vi "Lab Panel V5.0.vi"() -> ()   [LabVIEW 2013] (continued)
                  tunnel: w3944 -> [_ _ _ w4028 _]
                  tunnel: w3943 -> [_ _ _ w4027 _]
                  tunnel: w3942 -> [_ _ _ w4026 _]
                  tunnel: w3941 -> [_ _ _ w4025 _]
                  tunnel: w3940 -> [_ _ _ w4024 _]
                  tunnel: w3939 -> [_ _ _ w4023 _]
                  tunnel: w3938 -> [_ _ _ w4022 _]
                  frame #0 {
                    n2306 = Merge Signals(w3998, w3997, w3996, w3995, w3994, w3993, w3992, w3991, w3990, w3989) -> (→"TEST AMPS CHART":dynamicdata)
                  }
                  frame #1 {
                    n2307 = Merge Signals(w4009, w4008, w4007, w4006, w4005, w4004, w4003, w4002, w4001, w4000) -> (→"TEST VOLTS CHART":dynamicdata)
                  }
                  frame #2 {
                    n2308 = Merge Signals(w4020, w4019, w4018, w4017, w4016, w4015, w4014, w4013, w4012, w4011) -> (→"TEMPERATURE (L) CHART":dynamicdata)
                  }
                  frame #3 {
                    n2309 = Merge Signals(w4031, w4030, w4029, w4028, w4027, w4026, w4025, w4024, w4023, w4022) -> (→"TEMPERATURE (N) CHART":dynamicdata)
                  }
                  frame #4 {
                    n2310 = local read "TEMPERATURE (N) CHART"() -> (w4032:dynamicdata)
                    n2311 = local read "TEMPERATURE (L) CHART"() -> (w4033:dynamicdata)
                    n2312 = local read "TEST VOLTS CHART"() -> (w4034:dynamicdata)
                    n2313 = local read "TEST AMPS CHART"() -> (w4035:dynamicdata)
                    n2314 = global write "Global display 3.vi" "graph temp N"(w4032) -> ()
                    n2315 = global write "Global display 3.vi" "graph temp L"(w4033) -> ()
                    n2316 = global write "Global display 3.vi" "graph volts"(w4034) -> ()
                    n2317 = global write "Global display 3.vi" "graph amps"(w4035) -> ()
                  }
                }
              }
            }
          }
          frame #14 {
            # "check for amps fail"
            # "check for cycle test & temperature rise fail conditions"
            n2318 = local read "on loops"() -> (w4062:dbl)
            n2319 = local read "jig cycle"() -> (w4059:dbl)
            n2320 = local read "jig cycle"() -> (w4064:dbl)
            n2321 = Add(x=w4062, y=3.0) -> (x+y=w4060:dbl)
            n2322 = Equal?(x=w4059, y=w4060) -> (x = y?=w4055:bool)
            n2323 = local read "Fail Loops"() -> (w4036:dbl)
            n2324 = Equal?(x=w4064, y=1.0) -> (x = y?=w4057:bool)
            n2325 = global write "Global 1.vi" "fail count"(w4036) -> ()
            n2326 = stacked-sequence {
              tunnel: w4058 -> [w4067 _ _ _ _ _ _ _ _ _]
              tunnel: w4057 -> [w4068 w4088 w4108 w4128 w4148 w4168 w4188 w4208 w4228 w4248]
              tunnel: w4056 -> [w4065 _ _ _ _ _ _ _ _ _]
              tunnel: w4055 -> [w4066 w4087 w4107 w4127 w4147 w4167 w4187 w4207 w4227 w4247]
              tunnel: w4054 -> [_ w4086 _ _ _ _ _ _ _ _]
              tunnel: w4053 -> [_ w4085 _ _ _ _ _ _ _ _]
              tunnel: w4052 -> [_ _ w4106 _ _ _ _ _ _ _]
              tunnel: w4051 -> [_ _ w4105 _ _ _ _ _ _ _]
              tunnel: w4050 -> [_ _ _ w4126 _ _ _ _ _ _]
              tunnel: w4049 -> [_ _ _ w4125 _ _ _ _ _ _]
              tunnel: w4048 -> [_ _ _ _ w4146 _ _ _ _ _]
              tunnel: w4047 -> [_ _ _ _ w4145 _ _ _ _ _]
              tunnel: w4046 -> [_ _ _ _ _ w4166 _ _ _ _]
              tunnel: w4045 -> [_ _ _ _ _ w4165 _ _ _ _]
              tunnel: w4044 -> [_ _ _ _ _ _ w4186 _ _ _]
              tunnel: w4043 -> [_ _ _ _ _ _ w4185 _ _ _]
              tunnel: w4042 -> [_ _ _ _ _ _ _ w4206 _ _]
              tunnel: w4041 -> [_ _ _ _ _ _ _ w4205 _ _]
              tunnel: w4040 -> [_ _ _ _ _ _ _ _ w4226 _]
              tunnel: w4039 -> [_ _ _ _ _ _ _ _ w4225 _]
              tunnel: w4038 -> [_ _ _ _ _ _ _ _ _ w4246]
              tunnel: w4037 -> [_ _ _ _ _ _ _ _ _ w4245]
              frame #0 {
                # "LAB01-1"
                n2327 = case shown="True" w4065 {
                  tunnel: w4068 -> [_ w4081]
                  tunnel: w4067 -> [_ w4078]
                  tunnel: w4066 -> [_ w4077]
                  frame False {
                  }
                  frame True {
                    n2328 = local read "TEMP START LAB01-1"() -> (w4083:cluster{"TL":dbl, "TN":dbl})
                    n2329 = local read "RESULT LAB01-1"() -> (w4072:bool)
                    n2330 = local read "FAIL LAB01-1"() -> (w4075:cluster{"LO":dbl, "HI":dbl})
                    n2331 = local read "TDMS LAB01-1"() -> (w4082:refnum<k34>)
                    n2332 = local read "SET LAB01-1"() -> (w4079:T5)
                    n2333 = local read "DISP LAB01-1"() -> (w4080:T4)
                    n2334 = local read "SIG LAB01-1"() -> (w4084:T2)
                    n2335 = Bundle("FAIL LAB01-1"=w4075, "SIG LAB01-1"=w4084, "TEMP START LAB01-1"=w4083, "DISP LAB01-1"=w4080, "SET LAB01-1"=w4079, "TDMS LAB01-1"=w4082) -> (w4069:T28)  [unwired: 1 in]
                    n2336 = call "sub vi - cycle&temp fail v6.vi"("Amps Lo?"=w4081, "Input Cluster"=w4069, "SELECT"=w4078, "Amps Hi?"=w4077, "Result In"=w4072) -> ("(FAIL) out"=w4074:cluster{"FAIL LO":dbl, "FAIL HI":dbl}, "(DISP) out"=w4070:T4, "T-RISE"=w4071:cluster{"T-RISE (L)":dbl, "T-RISE (N)":dbl}, "Result Out"=w4073:bool, "file error"=w4076:errorcluster)  [unwired: 10 in]
                    n2337 = local write "TEMP RISE LAB01-1"(w4071) -> ()
                    n2338 = local write "FAIL LAB01-1"(w4074) -> ()
                    n2339 = local write "DISP LAB01-1"(w4070) -> ()
                    n2340 = local write "RESULT LAB01-1"(w4073) -> ()
                    n2341 = local write "data file error"(w4076) -> ()
                  }
                }
              }
              frame #1 {
                # "LAB01-2"
                n2342 = case shown="True" w4086 {
                  tunnel: w4088 -> [_ w4101]
                  tunnel: w4085 -> [_ w4098]
                  tunnel: w4087 -> [_ w4097]
                  frame False {
                  }
                  frame True {
                    n2343 = local read "TEMP START LAB01-2"() -> (w4103:cluster{"TL":dbl, "TN":dbl})
                    n2344 = local read "FAIL LAB01-2"() -> (w4094:cluster{"LO":dbl, "HI":dbl})
                    n2345 = local read "TDMS LAB01-2"() -> (w4102:refnum<k34>)
                    n2346 = local read "SET LAB01-2"() -> (w4099:T5)
                    n2347 = local read "DISP LAB01-2"() -> (w4100:T4)
                    n2348 = local read "RESULT LAB01-2"() -> (w4091:bool)
                    n2349 = local read "SIG LAB01-2"() -> (w4104:T2)
                    n2350 = Bundle("FAIL LAB01-2"=w4094, "SIG LAB01-2"=w4104, "TEMP START LAB01-2"=w4103, "DISP LAB01-2"=w4100, "SET LAB01-2"=w4099, "TDMS LAB01-2"=w4102) -> (w4089:T29)  [unwired: 1 in]
                    n2351 = call "sub vi - cycle&temp fail v6.vi"("Amps Lo?"=w4101, "Input Cluster"=w4089, "SELECT"=w4098, "Amps Hi?"=w4097, "Result In"=w4091) -> ("(FAIL) out"=w4093:cluster{"FAIL LO":dbl, "FAIL HI":dbl}, "(DISP) out"=w4096:T4, "T-RISE"=w4090:cluster{"T-RISE (L)":dbl, "T-RISE (N)":dbl}, "Result Out"=w4092:bool, "file error"=w4095:errorcluster)  [unwired: 10 in]
                    n2352 = local write "TEMP RISE LAB01-2"(w4090) -> ()
                    n2353 = local write "FAIL LAB01-2"(w4093) -> ()
                    n2354 = local write "DISP LAB01-2"(w4096) -> ()
                    n2355 = local write "RESULT LAB01-2"(w4092) -> ()
                    n2356 = local write "data file error"(w4095) -> ()
                  }
                }
              }
              frame #2 {
                # "LAB02-1"
                n2357 = case shown="True" w4106 {
                  tunnel: w4108 -> [_ w4121]
                  tunnel: w4105 -> [_ w4118]
                  tunnel: w4107 -> [_ w4117]
                  frame False {
                  }
                  frame True {
                    n2358 = local read "TEMP START LAB02-1"() -> (w4123:cluster{"TL":dbl, "TN":dbl})
                    n2359 = local read "FAIL LAB02-1"() -> (w4114:cluster{"LO":dbl, "HI":dbl})
                    n2360 = local read "TDMS LAB02-1"() -> (w4122:refnum<k34>)
                    n2361 = local read "SET LAB02-1"() -> (w4119:T5)
                    n2362 = local read "DISP LAB02-1"() -> (w4120:T4)
                    n2363 = local read "SIG LAB02-1"() -> (w4124:T2)
                    n2364 = local read "RESULT LAB02-1"() -> (w4111:bool)
                    n2365 = Bundle("FAIL LAB02-1"=w4114, "SIG LAB02-1"=w4124, "TEMP START LAB02-1"=w4123, "DISP LAB02-1"=w4120, "SET LAB02-1"=w4119, "TDMS LAB02-1"=w4122) -> (w4109:T30)  [unwired: 1 in]
                    n2366 = call "sub vi - cycle&temp fail v6.vi"("Amps Lo?"=w4121, "Input Cluster"=w4109, "SELECT"=w4118, "Amps Hi?"=w4117, "Result In"=w4111) -> ("(FAIL) out"=w4113:cluster{"FAIL LO":dbl, "FAIL HI":dbl}, "(DISP) out"=w4116:T4, "T-RISE"=w4110:cluster{"T-RISE (L)":dbl, "T-RISE (N)":dbl}, "Result Out"=w4112:bool, "file error"=w4115:errorcluster)  [unwired: 10 in]
                    n2367 = local write "TEMP RISE LAB02-1"(w4110) -> ()
                    n2368 = local write "FAIL LAB02-1"(w4113) -> ()
                    n2369 = local write "DISP LAB02-1"(w4116) -> ()
                    n2370 = local write "RESULT LAB02-1"(w4112) -> ()
                    n2371 = local write "data file error"(w4115) -> ()
                  }
                }
              }
              frame #3 {
                # "LAB02-2"
                n2372 = case shown="True" w4126 {
                  tunnel: w4128 -> [_ w4141]
                  tunnel: w4125 -> [_ w4138]
                  tunnel: w4127 -> [_ w4137]
                  frame False {
                  }
                  frame True {
                    n2373 = local read "TEMP START LAB02-2"() -> (w4143:cluster{"TL":dbl, "TN":dbl})
                    n2374 = local read "FAIL LAB02-2"() -> (w4134:cluster{"LO":dbl, "HI":dbl})
                    n2375 = local read "TDMS LAB02-2"() -> (w4142:refnum<k34>)
                    n2376 = local read "SET LAB02-2"() -> (w4139:T5)
                    n2377 = local read "DISP LAB02-2"() -> (w4140:T4)
                    n2378 = local read "SIG LAB02-2"() -> (w4144:T2)
                    n2379 = local read "RESULT LAB02-2"() -> (w4131:bool)
                    n2380 = Bundle("FAIL LAB02-2"=w4134, "SIG LAB02-2"=w4144, "TEMP START LAB02-2"=w4143, "DISP LAB02-2"=w4140, "SET LAB02-2"=w4139, "TDMS LAB02-2"=w4142) -> (w4129:T31)  [unwired: 1 in]
                    n2381 = call "sub vi - cycle&temp fail v6.vi"("Amps Lo?"=w4141, "Input Cluster"=w4129, "SELECT"=w4138, "Amps Hi?"=w4137, "Result In"=w4131) -> ("(FAIL) out"=w4133:cluster{"FAIL LO":dbl, "FAIL HI":dbl}, "(DISP) out"=w4136:T4, "T-RISE"=w4130:cluster{"T-RISE (L)":dbl, "T-RISE (N)":dbl}, "Result Out"=w4132:bool, "file error"=w4135:errorcluster)  [unwired: 10 in]
                    n2382 = local write "TEMP RISE LAB02-2"(w4130) -> ()
                    n2383 = local write "FAIL LAB02-2"(w4133) -> ()
                    n2384 = local write "DISP LAB02-2"(w4136) -> ()
                    n2385 = local write "RESULT LAB02-2"(w4132) -> ()
                    n2386 = local write "data file error"(w4135) -> ()
                  }
                }
              }
              frame #4 {
                # "LAB03-1"
                n2387 = case shown="True" w4146 {
                  tunnel: w4148 -> [_ w4161]
                  tunnel: w4145 -> [_ w4158]
                  tunnel: w4147 -> [_ w4157]
                  frame False {
                  }
                  frame True {
                    n2388 = local read "TEMP START LAB03-1"() -> (w4163:cluster{"TL":dbl, "TN":dbl})
                    n2389 = local read "FAIL LAB03-1"() -> (w4154:cluster{"LO":dbl, "HI":dbl})
                    n2390 = local read "TDMS LAB03-1"() -> (w4162:refnum<k34>)
                    n2391 = local read "SET LAB03-1"() -> (w4159:T5)
                    n2392 = local read "DISP LAB03-1"() -> (w4160:T4)
                    n2393 = local read "SIG LAB03-1"() -> (w4164:T2)
                    n2394 = local read "RESULT LAB03-1"() -> (w4151:bool)
                    n2395 = Bundle("FAIL LAB03-1"=w4154, "SIG LAB03-1"=w4164, "TEMP START LAB03-1"=w4163, "DISP LAB03-1"=w4160, "SET LAB03-1"=w4159, "TDMS LAB03-1"=w4162) -> (w4149:T32)  [unwired: 1 in]
                    n2396 = call "sub vi - cycle&temp fail v6.vi"("Amps Lo?"=w4161, "Input Cluster"=w4149, "SELECT"=w4158, "Amps Hi?"=w4157, "Result In"=w4151) -> ("(FAIL) out"=w4153:cluster{"FAIL LO":dbl, "FAIL HI":dbl}, "(DISP) out"=w4156:T4, "T-RISE"=w4150:cluster{"T-RISE (L)":dbl, "T-RISE (N)":dbl}, "Result Out"=w4152:bool, "file error"=w4155:errorcluster)  [unwired: 10 in]
                    n2397 = local write "TEMP RISE LAB03-1"(w4150) -> ()
                    n2398 = local write "FAIL LAB03-1"(w4153) -> ()
                    n2399 = local write "DISP LAB03-1"(w4156) -> ()
                    n2400 = local write "RESULT LAB03-1"(w4152) -> ()
                    n2401 = local write "data file error"(w4155) -> ()
                  }
                }
              }
              frame #5 {
                # "LAB03-2"
                n2402 = case shown="True" w4166 {
                  tunnel: w4168 -> [_ w4181]
                  tunnel: w4165 -> [_ w4178]
                  tunnel: w4167 -> [_ w4177]
                  frame False {
                  }
                  frame True {
                    n2403 = local read "TEMP START LAB03-2"() -> (w4183:cluster{"TL":dbl, "TN":dbl})
                    n2404 = local read "FAIL LAB03-2"() -> (w4174:cluster{"LO":dbl, "HI":dbl})
                    n2405 = local read "TDMS LAB03-2"() -> (w4182:refnum<k34>)
                    n2406 = local read "SET LAB03-2"() -> (w4179:T5)
                    n2407 = local read "DISP LAB03-2"() -> (w4180:T4)
                    n2408 = local read "RESULT LAB03-2"() -> (w4171:bool)
                    n2409 = local read "SIG LAB03-2"() -> (w4184:T2)
                    n2410 = Bundle("FAIL LAB03-2"=w4174, "SIG LAB03-2"=w4184, "TEMP START LAB03-2"=w4183, "DISP LAB03-2"=w4180, "SET LAB03-2"=w4179, "TDMS LAB03-2"=w4182) -> (w4169:T33)  [unwired: 1 in]
                    n2411 = call "sub vi - cycle&temp fail v6.vi"("Amps Lo?"=w4181, "Input Cluster"=w4169, "SELECT"=w4178, "Amps Hi?"=w4177, "Result In"=w4171) -> ("(FAIL) out"=w4173:cluster{"FAIL LO":dbl, "FAIL HI":dbl}, "(DISP) out"=w4176:T4, "T-RISE"=w4170:cluster{"T-RISE (L)":dbl, "T-RISE (N)":dbl}, "Result Out"=w4172:bool, "file error"=w4175:errorcluster)  [unwired: 10 in]
                    n2412 = local write "FAIL LAB03-2"(w4173) -> ()
                    n2413 = local write "TEMP RISE LAB03-2"(w4170) -> ()
                    n2414 = local write "DISP LAB03-2"(w4176) -> ()
                    n2415 = local write "RESULT LAB03-2"(w4172) -> ()
                    n2416 = local write "data file error"(w4175) -> ()
                  }
                }
              }
              frame #6 {
                # "LAB04-1"
                n2417 = case shown="True" w4186 {
                  tunnel: w4188 -> [_ w4201]
                  tunnel: w4185 -> [_ w4198]
                  tunnel: w4187 -> [_ w4197]
                  frame False {
                  }
                  frame True {
                    n2418 = local read "TEMP START LAB04-1"() -> (w4203:cluster{"TL":dbl, "TN":dbl})
                    n2419 = local read "FAIL LAB04-1"() -> (w4194:cluster{"LO":dbl, "HI":dbl})
                    n2420 = local read "TDMS LAB04-1"() -> (w4202:refnum<k34>)
                    n2421 = local read "SET LAB04-1"() -> (w4199:T5)
                    n2422 = local read "DISP LAB04-1"() -> (w4200:T4)
                    n2423 = local read "SIG LAB04-1"() -> (w4204:T2)
                    n2424 = local read "RESULT LAB04-1"() -> (w4191:bool)
                    n2425 = Bundle("FAIL LAB04-1"=w4194, "SIG LAB04-1"=w4204, "TEMP START LAB04-1"=w4203, "DISP LAB04-1"=w4200, "SET LAB04-1"=w4199, "TDMS LAB04-1"=w4202) -> (w4189:T34)  [unwired: 1 in]
                    n2426 = call "sub vi - cycle&temp fail v6.vi"("Amps Lo?"=w4201, "Input Cluster"=w4189, "SELECT"=w4198, "Amps Hi?"=w4197, "Result In"=w4191) -> ("(FAIL) out"=w4193:cluster{"FAIL LO":dbl, "FAIL HI":dbl}, "(DISP) out"=w4196:T4, "T-RISE"=w4190:cluster{"T-RISE (L)":dbl, "T-RISE (N)":dbl}, "Result Out"=w4192:bool, "file error"=w4195:errorcluster)  [unwired: 10 in]
                    n2427 = local write "TEMP RISE LAB04-1"(w4190) -> ()
                    n2428 = local write "FAIL LAB04-1"(w4193) -> ()
                    n2429 = local write "DISP LAB04-1"(w4196) -> ()
                    n2430 = local write "RESULT LAB04-1"(w4192) -> ()
                    n2431 = local write "data file error"(w4195) -> ()
                  }
                }
              }
              frame #7 {
                # "LAB04-2"
                n2432 = case shown="True" w4206 {
                  tunnel: w4208 -> [_ w4221]
                  tunnel: w4205 -> [_ w4218]
                  tunnel: w4207 -> [_ w4217]
                  frame False {
                  }
                  frame True {
                    n2433 = local read "TEMP START LAB04-2"() -> (w4223:cluster{"TL":dbl, "TN":dbl})
                    n2434 = local read "FAIL LAB04-2"() -> (w4214:cluster{"LO":dbl, "HI":dbl})
                    n2435 = local read "TDMS LAB04-2"() -> (w4222:refnum<k34>)
                    n2436 = local read "SET LAB04-2"() -> (w4219:T5)
                    n2437 = local read "DISP LAB04-2"() -> (w4220:T4)
                    n2438 = local read "SIG LAB04-2"() -> (w4224:T2)
                    n2439 = local read "RESULT LAB04-2"() -> (w4211:bool)
                    n2440 = Bundle("FAIL LAB04-2"=w4214, "SIG LAB04-2"=w4224, "TEMP START LAB04-2"=w4223, "DISP LAB04-2"=w4220, "SET LAB04-2"=w4219, "TDMS LAB04-2"=w4222) -> (w4209:T35)  [unwired: 1 in]
                    n2441 = call "sub vi - cycle&temp fail v6.vi"("Amps Lo?"=w4221, "Input Cluster"=w4209, "SELECT"=w4218, "Amps Hi?"=w4217, "Result In"=w4211) -> ("(FAIL) out"=w4213:cluster{"FAIL LO":dbl, "FAIL HI":dbl}, "(DISP) out"=w4216:T4, "T-RISE"=w4210:cluster{"T-RISE (L)":dbl, "T-RISE (N)":dbl}, "Result Out"=w4212:bool, "file error"=w4215:errorcluster)  [unwired: 10 in]
                    n2442 = local write "TEMP RISE LAB04-2"(w4210) -> ()
                    n2443 = local write "FAIL LAB04-2"(w4213) -> ()
                    n2444 = local write "DISP LAB04-2"(w4216) -> ()
                    n2445 = local write "RESULT LAB04-2"(w4212) -> ()
                    n2446 = local write "data file error"(w4215) -> ()
                  }
                }
              }
              frame #8 {
                # "LAB05-1"
                n2447 = case shown="True" w4226 {
                  tunnel: w4228 -> [_ w4241]
                  tunnel: w4225 -> [_ w4238]
                  tunnel: w4227 -> [_ w4237]
                  frame False {
                  }
                  frame True {
                    n2448 = local read "TEMP START LAB05-1"() -> (w4243:cluster{"TL":dbl, "TN":dbl})
                    n2449 = local read "FAIL LAB05-1"() -> (w4234:cluster{"LO":dbl, "HI":dbl})
                    n2450 = local read "TDMS LAB05-1"() -> (w4242:refnum<k34>)
                    n2451 = local read "SET LAB05-1"() -> (w4239:T5)
                    n2452 = local read "DISP LAB05-1"() -> (w4240:T4)
                    n2453 = local read "SIG LAB05-1"() -> (w4244:T2)
                    n2454 = local read "RESULT LAB05-1"() -> (w4231:bool)
                    n2455 = Bundle("FAIL LAB05-1"=w4234, "SIG LAB05-1"=w4244, "TEMP START LAB05-1"=w4243, "DISP LAB05-1"=w4240, "SET LAB05-1"=w4239, "TDMS LAB05-1"=w4242) -> (w4229:T36)  [unwired: 1 in]
                    n2456 = call "sub vi - cycle&temp fail v6.vi"("Amps Lo?"=w4241, "Input Cluster"=w4229, "SELECT"=w4238, "Amps Hi?"=w4237, "Result In"=w4231) -> ("(FAIL) out"=w4233:cluster{"FAIL LO":dbl, "FAIL HI":dbl}, "(DISP) out"=w4236:T4, "T-RISE"=w4230:cluster{"T-RISE (L)":dbl, "T-RISE (N)":dbl}, "Result Out"=w4232:bool, "file error"=w4235:errorcluster)  [unwired: 10 in]
                    n2457 = local write "TEMP RISE LAB05-1"(w4230) -> ()
                    n2458 = local write "FAIL LAB05-1"(w4233) -> ()
                    n2459 = local write "DISP LAB05-1"(w4236) -> ()
                    n2460 = local write "RESULT LAB05-1"(w4232) -> ()
                    n2461 = local write "data file error"(w4235) -> ()
                  }
                }
              }
              frame #9 {
                # "LAB05-2"
                n2462 = case shown="True" w4246 {
                  tunnel: w4248 -> [_ w4261]
                  tunnel: w4245 -> [_ w4258]
                  tunnel: w4247 -> [_ w4257]
                  frame False {
                  }
                  frame True {
                    n2463 = local read "TEMP START LAB05-2"() -> (w4263:cluster{"TL":dbl, "TN":dbl})
                    n2464 = local read "FAIL LAB05-2"() -> (w4254:cluster{"LO":dbl, "HI":dbl})
                    n2465 = local read "TDMS LAB05-2"() -> (w4262:refnum<k34>)
                    n2466 = local read "SET LAB05-2"() -> (w4259:T5)
                    n2467 = local read "DISP LAB05-2"() -> (w4260:T4)
                    n2468 = local read "SIG LAB05-2"() -> (w4264:T2)
                    n2469 = local read "RESULT LAB05-2"() -> (w4251:bool)
                    n2470 = Bundle("FAIL LAB05-2"=w4254, "SIG LAB05-2"=w4264, "TEMP START LAB05-2"=w4263, "DISP LAB05-2"=w4260, "SET LAB05-2"=w4259, "TDMS LAB05-2"=w4262) -> (w4249:T37)  [unwired: 1 in]
                    n2471 = call "sub vi - cycle&temp fail v6.vi"("Amps Lo?"=w4261, "Input Cluster"=w4249, "SELECT"=w4258, "Amps Hi?"=w4257, "Result In"=w4251) -> ("(FAIL) out"=w4253:cluster{"FAIL LO":dbl, "FAIL HI":dbl}, "(DISP) out"=w4256:T4, "T-RISE"=w4250:cluster{"T-RISE (L)":dbl, "T-RISE (N)":dbl}, "Result Out"=w4252:bool, "file error"=w4255:errorcluster)  [unwired: 10 in]
                    n2472 = local write "TEMP RISE LAB05-2"(w4250) -> ()
                    n2473 = local write "FAIL LAB05-2"(w4253) -> ()
                    n2474 = local write "DISP LAB05-2"(w4256) -> ()
                    n2475 = local write "RESULT LAB05-2"(w4252) -> ()
                    n2476 = local write "data file error"(w4255) -> ()
                  }
                }
              }
            }
          }
          frame #15 {
            # "run calibration routine"
            n2477 = local read "SET (cal)"() -> (w4265:bool)
            n2478 = case shown="True" w4265 {
              frame False {
              }
              frame True {
                n2479 = stacked-sequence {
                  seq-local: [w4266 _ _] -> [_ w4268 _]
                  frame #0 {
                    n2480 = call "CALIBRATION PASSWORD"() -> ("PASSWORD"=w4266:string)  [unwired: 17 in, 2 out]
                  }
                  frame #1 {
                    n2481 = Equal?(x=w4268, y="7777") -> (x = y?=w4267:bool)
                    n2482 = case shown="True" w4267 {
                      frame False {
                      }
                      frame True {
                        n2483 = stacked-sequence {
                          frame #0 {
                            n2484 = call "sub vi - calibration v1.vi"() -> ()  [unwired: 12 in]
                          }
                          frame #1 {
                            n2485 = call "sub vi - get calibration values v1.vi"() -> ("LAB01 (CAL)"=w4274:T12, "LAB02 (CAL)"=w4273:T13, "LAB03 (CAL)"=w4272:T12, "LAB04 (CAL)"=w4271:T12, "calibration file error out"=w4275:errorcluster, "LAB05 (CAL)"=w4270:T12)  [unwired: 9 in, 1 out]
                            n2486 = local write "cal file error out"(w4275) -> ()
                            n2487 = local write "CAL LAB04"(w4271) -> ()
                            n2488 = local write "CAL LAB05"(w4270) -> ()
                            n2489 = local write "CAL LAB01"(w4274) -> ()
                            n2490 = local write "CAL LAB02"(w4273) -> ()
                            n2491 = local write "CAL LAB03"(w4272) -> ()
                          }
                        }
                      }
                    }
                  }
                  frame #2 {
                    n2492 = local write "SET (cal)"(FALSE) -> ()
                  }
                }
              }
            }
          }
          frame #16 {
            # "save certain settings to file"
            n2493 = String To Path(string="c:\\crabtree\\Set Up\\") -> (path=w4278:path)
            n2494 = Build Path(base path=w4278, name or relative path="settings.bin") -> (appended path=w4280:path)
            n2495 = Build Path(base path=w4278, name or relative path="mail.bin") -> (appended path=w4277:path)
            n2496 = Create Folder(path (use dialog)=w4278) -> (error out=w4283:errorcluster)  [unwired: 2 in, 2 out]
            n2497 = call <vilib>:"Clear Errors.vi"("error in (no error)"=w4283) -> ()  [unwired: 6 in, 1 out]
            n2498 = stacked-sequence {
              seq-local: [w4293 _] -> [_ w4306]
              tunnel: w4280 -> [_ w4307]
              tunnel: w4277 -> [_ w4305]
              frame #0 {
                n2499 = local read "C drive data root dir"() -> (w4292:path)
                n2500 = local read "Select COM port"() -> (w4289:refnum<visa-resource-name>)
                n2501 = local read "Network Directory"() -> (w4298:path)
                n2502 = local read "SET LAB05-2"() -> (w4297:T5)
                n2503 = local read "SET LAB05-1"() -> (w4296:T5)
                n2504 = local read "SET LAB04-2"() -> (w4295:T5)
                n2505 = local read "SET LAB03-2"() -> (w4299:T5)
                n2506 = local read "SET LAB04-1"() -> (w4294:T5)
                n2507 = local read "SET LAB03-1"() -> (w4300:T5)
                n2508 = local read "SET LAB02-2"() -> (w4301:T5)
                n2509 = local read "SET LAB02-1"() -> (w4302:T5)
                n2510 = local read "Temp Delay Lps"() -> (w4288:dbl)
                n2511 = local read "SET LAB01-2"() -> (w4303:T5)
                n2512 = local read "Temp Test Cal"() -> (w4285:dbl)
                n2513 = local read "SET LAB01-1"() -> (w4304:T5)
                n2514 = local read "Temp Value"() -> (w4287:dbl)
                n2515 = local read "Fail Loops"() -> (w4286:dbl)
                n2516 = local read "spare"() -> (w4284:dbl)
                n2517 = local read "RATE (Hz)"() -> (w4291:dbl)
                n2518 = local read "SAMPLES"() -> (w4290:dbl)
                n2519 = Bundle("SET LAB01-1"=w4304, "SET LAB01-2"=w4303, "SET LAB02-1"=w4302, "SET LAB02-2"=w4301, "SET LAB03-1"=w4300, "SET LAB03-2"=w4299, "SET LAB04-1"=w4294, "SET LAB04-2"=w4295, "SET LAB05-1"=w4296, "SET LAB05-2"=w4297, "Network Directory"=w4298, "C drive data root dir"=w4292, "RATE (Hz)"=w4291, "SAMPLES"=w4290, "Select COM port"=w4289, "Temp Delay Lps"=w4288, "Temp Value"=w4287, "Fail Loops"=w4286, "Temp Test Cal"=w4285, "spare"=w4284) -> (w4293:T20)  [unwired: 1 in]
              }
              frame #1 {
                n2520 = event shown="[1] \"SET LAB01-1\", \"SET LAB01-2\", \"SET LAB02-1\", \"SET LAB02-2\", \"SET LAB03-1\", \"SET LAB03-2\", \"SET LAB04-1\", \"SET LAB04-2\", \"SET LAB05-1\", \"SET LAB05-2\", \"Network Directory\", \"C drive data root dir\", \"RATE (Hz)\", \"SAMPLES\", \"Select COM port\", \"Temp Delay Lps\", \"Temp Value\", \"Fail Loops\", \"Temp Test Cal\", \"spare\": Value Change" {
                  selector: _ -> [_ _ _]
                  dyn-events: _ -> [_ _ _]
                  timeout: 10.0 -> [_ _ _]
                  tunnel: w4307 -> [_ w4309 _]
                  tunnel: w4306 -> [_ w4310 _]
                  tunnel: w4305 -> [_ _ w4321]
                  event Timeout {
                    n2521 = event-data() -> ()  [unwired: 1 in, 3 out]
                  }
                  event "SET LAB01-1", "SET LAB01-2", "SET LAB02-1", "SET LAB02-2", "SET LAB03-1", "SET LAB03-2", "SET LAB04-1", "SET LAB04-2", "SET LAB05-1", "SET LAB05-2", "Network Directory", "C drive data root dir", "RATE (Hz)", "SAMPLES", "Select COM port", "Temp Delay Lps", "Temp Value", "Fail Loops", "Temp Test Cal", "spare": Value Change {
                    n2522 = event-data() -> ()  [unwired: 1 in, 6 out]
                    n2523 = Open/Create/Replace File(file path (use dialog)=w4309, operation (0:open)=T19."replace or create") -> (refnum out=w4315:refnum<file>, error out=w4314:errorcluster)  [unwired: 4 in, 1 out]
                    n2524 = Write to Binary File(file (use dialog)=w4315, data=w4310, error in=w4314) -> (refnum out=w4313:refnum<file>, error out=w4312:errorcluster)  [unwired: 3 in, 1 out]
                    n2525 = Close File(refnum=w4313, error in=w4312) -> (error out=w4311:errorcluster)  [unwired: 1 out]
                    n2526 = local write "data file error"(w4311) -> ()
                  }
                  event "MAIL SETTINGS.OUT SERVER ADDRESS", "MAIL SETTINGS.FROM ACCOUNT", "MAIL SETTINGS.USER NAME", "MAIL SETTINGS.PASSWORD", "Auto Mail Send", "TO (string):": Value Change {
                    n2527 = event-data() -> ()  [unwired: 1 in, 6 out]
                    n2528 = local read "MAIL SETTINGS"() -> (w4320:T6)
                    n2529 = local read "Auto Mail Send"() -> (w4318:bool)
                    n2530 = local read "TO (string):"() -> (w4317:string)
                    n2531 = Open/Create/Replace File(file path (use dialog)=w4321, operation (0:open)=T19."replace or create") -> (refnum out=w4326:refnum<file>, error out=w4325:errorcluster)  [unwired: 4 in, 1 out]
                    n2532 = Bundle("MAIL SETTINGS"=w4320, "Auto Mail Send"=w4318, "TO (string):"=w4317) -> (w4319:T38)  [unwired: 1 in]
                    n2533 = Write to Binary File(file (use dialog)=w4326, data=w4319, error in=w4325) -> (refnum out=w4324:refnum<file>, error out=w4323:errorcluster)  [unwired: 3 in, 1 out]
                    n2534 = Close File(refnum=w4324, error in=w4323) -> (error out=w4322:errorcluster)  [unwired: 1 out]
                    n2535 = local write "data file error"(w4322) -> ()
                  }
                }
              }
            }
          }
          frame #17 {
            # "mail control"
            n2536 = local read "MAIL SETTINGS"() -> (w4343:T6)
            n2537 = local read "Auto Mail Send"() -> (w4329:bool)
            n2538 = Unbundle(w4343) -> ("OUT SERVER ADDRESS"=w4342:string, "FROM ACCOUNT"=w4341:string, "TEST MAIL"=w4340:bool)  [unwired: 4 out]
            n2539 = stacked-sequence {
              tunnel: "TO (string):" -> [_ w4382]
              tunnel: w4343 -> [w4348 w4381]
              tunnel: w4342 -> [w4347 w4380]
              tunnel: w4341 -> [w4346 w4379]
              tunnel: w4340 -> [w4345 _]
              tunnel: w4329 -> [_ w4378]
              tunnel: w4339 -> [_ w4377]
              tunnel: w4338 -> [_ w4376]
              tunnel: w4337 -> [_ w4375]
              tunnel: w4336 -> [_ w4374]
              tunnel: w4335 -> [_ w4373]
              tunnel: w4334 -> [_ w4372]
              tunnel: w4333 -> [_ w4371]
              tunnel: w4332 -> [_ w4370]
              tunnel: w4331 -> [_ w4369]
              tunnel: w4330 -> [_ w4368]
              tunnel: "TO (string):" -> [w4344 _]
              frame #0 {
                # "mail test"
                n2540 = case shown="True" w4345 {
                  tunnel: w4348 -> [_ w4352]
                  tunnel: w4344 -> [_ w4351]
                  tunnel: w4347 -> [_ w4350]
                  tunnel: w4346 -> [_ w4349]
                  frame False {
                  }
                  frame True {
                    n2541 = stacked-sequence {
                      seq-local: [_ _ w4362 _] -> [_ _ _ w4363]
                      tunnel: w4352 -> [w4355 _ _ w4367]
                      tunnel: w4351 -> [_ _ w4360 _]
                      tunnel: w4350 -> [_ _ w4358 _]
                      tunnel: w4349 -> [_ _ w4359 _]
                      frame #0 {
                        n2542 = Bundle(cluster=w4355, "TEST MAIL STATUS"="TEST START") -> (w4353:T6)  [unwired: 6 in]
                        n2543 = local write "MAIL SETTINGS"(w4353) -> ()
                      }
                      frame #1 {
                        n2544 = Wait (ms)(milliseconds to wait=500) -> ()  [unwired: 1 out]
                      }
                      frame #2 {
                        n2545 = call "sub vi - send mail with attach v5.vi"("TO:"=w4360, "subject"="MAIL TEST FROM LAB PANEL", "from"=w4359, "out going server"=w4358, "message"="TEST MESSAGE") -> ("error out"=w4362:errorcluster)  [unwired: 10 in]
                      }
                      frame #3 {
                        n2546 = Bundle(cluster=w4367, "TEST MAIL"=FALSE, "TEST MAIL STATUS"="TEST END", "mail error"=w4363) -> (w4365:T6)  [unwired: 4 in]
                        n2547 = local write "MAIL SETTINGS"(w4365) -> ()
                      }
                    }
                  }
                }
              }
              frame #1 {
                # "mail report"
                n2548 = stacked-sequence {
                  seq-local: [_ w4425 _ _] -> [_ _ _ w4615]
                  seq-local: [_ _ w4528 _] -> [_ _ _ w4605]
                  seq-local: [w4392 _ _ _] -> [_ w4442 _ _]
                  seq-local: [w4391 _ _ _] -> [_ w4441 _ _]
                  seq-local: [w4389 _ _ _] -> [_ w4439 _ _]
                  seq-local: [w4390 _ _ _] -> [_ w4440 _ _]
                  seq-local: [w4388 _ _ _] -> [_ w4438 _ _]
                  seq-local: [w4387 _ _ _] -> [_ w4433 _ _]
                  seq-local: [w4386 _ _ _] -> [_ w4434 _ _]
                  seq-local: [w4385 _ _ _] -> [_ w4435 _ _]
                  seq-local: [w4384 _ _ _] -> [_ w4436 _ _]
                  seq-local: [w4383 _ _ _] -> [_ w4437 _ _]
                  tunnel: w4382 -> [_ _ _ w4616]
                  tunnel: w4381 -> [_ _ _ w4599]
                  tunnel: w4380 -> [_ _ _ w4613]
                  tunnel: w4379 -> [_ _ _ w4612]
                  tunnel: w4378 -> [w4423 _ _ w4607]
                  tunnel: w4377 -> [_ _ w4558 _]
                  tunnel: w4376 -> [_ _ w4555 _]
                  tunnel: w4375 -> [_ _ w4554 _]
                  tunnel: w4374 -> [_ _ w4553 _]
                  tunnel: w4373 -> [_ _ w4552 _]
                  tunnel: w4372 -> [_ _ w4551 _]
                  tunnel: w4371 -> [_ _ w4550 _]
                  tunnel: w4370 -> [_ _ w4549 _]
                  tunnel: w4369 -> [_ _ w4548 _]
                  tunnel: w4368 -> [_ _ w4547 _]
                  frame #0 {
                    n2549 = case shown="False" w4423 {
                      frame False {
                        n2550 = local write "mail control"("") -> ()
                      }
                      frame True {
                      }
                    }
                    n2551 = local read "SET LAB01-1"() -> (w4422:T5)
                    n2552 = local read "SET LAB01-2"() -> (w4421:T5)
                    n2553 = local read "SET LAB02-1"() -> (w4420:T5)
                    n2554 = local read "SET LAB02-2"() -> (w4419:T5)
                    n2555 = local read "SET LAB03-1"() -> (w4418:T5)
                    n2556 = local read "SET LAB04-1"() -> (w4416:T5)
                    n2557 = local read "SET LAB05-1"() -> (w4414:T5)
                    n2558 = local read "SET LAB03-2"() -> (w4417:T5)
                    n2559 = local read "SET LAB04-2"() -> (w4415:T5)
                    n2560 = local read "SET LAB05-2"() -> (w4413:T5)
                    n2561 = Unbundle(w4418) -> ("DESCRIPTION"=w4398:string)  [unwired: 4 out]
                    n2562 = Unbundle(w4417) -> ("DESCRIPTION"=w4397:string)  [unwired: 4 out]
                    n2563 = Unbundle(w4416) -> ("DESCRIPTION"=w4396:string)  [unwired: 4 out]
                    n2564 = Unbundle(w4413) -> ("DESCRIPTION"=w4393:string)  [unwired: 4 out]
                    n2565 = Unbundle(w4419) -> ("DESCRIPTION"=w4399:string)  [unwired: 4 out]
                    n2566 = Unbundle(w4415) -> ("DESCRIPTION"=w4395:string)  [unwired: 4 out]
                    n2567 = Unbundle(w4422) -> ("DESCRIPTION"=w4411:string)  [unwired: 4 out]
                    n2568 = Unbundle(w4420) -> ("DESCRIPTION"=w4400:string)  [unwired: 4 out]
                    n2569 = Unbundle(w4414) -> ("DESCRIPTION"=w4394:string)  [unwired: 4 out]
                    n2570 = Unbundle(w4421) -> ("DESCRIPTION"=w4401:string)  [unwired: 4 out]
                    n2571 = Concatenate Strings("[LAB05-2/", w4393) -> (w4383:string)
                    n2572 = Concatenate Strings("[LAB05-1/", w4394) -> (w4384:string)
                    n2573 = Concatenate Strings("[LAB04-2/", w4395) -> (w4385:string)
                    n2574 = Concatenate Strings("[LAB03-2/", w4397) -> (w4387:string)
                    n2575 = Concatenate Strings("[LAB04-1/", w4396) -> (w4386:string)
                    n2576 = Concatenate Strings("[LAB03-1/", w4398) -> (w4388:string)
                    n2577 = Concatenate Strings("[LAB01-2/", w4401) -> (w4391:string)
                    n2578 = Concatenate Strings("[LAB02-2/", w4399) -> (w4389:string)
                    n2579 = Concatenate Strings("[LAB01-1/", w4411) -> (w4392:string)
                    n2580 = Concatenate Strings("[LAB02-1/", w4400) -> (w4390:string)
                  }
                  frame #1 {
                    w4446 = "/"
                    w4447 = 2.0
                    n2581 = local read "DISP LAB01-2"() -> (w4526:T4)
                    n2582 = local read "DISP LAB01-1"() -> (w4527:T4)
                    n2583 = local read "DISP LAB02-1"() -> (w4525:T4)
                    n2584 = local read "DISP LAB03-2"() -> (w4522:T4)
                    n2585 = local read "DISP LAB02-2"() -> (w4524:T4)
                    n2586 = local read "DISP LAB03-1"() -> (w4523:T4)
                    n2587 = local read "DISP LAB04-2"() -> (w4520:T4)
                    n2588 = local read "DISP LAB04-1"() -> (w4521:T4)
                    n2589 = local read "DISP LAB05-1"() -> (w4519:T4)
                    n2590 = local read "DISP LAB05-2"() -> (w4518:T4)
                    n2591 = Unbundle(w4526) -> ("CYCLE"=w4510:dbl, "MINS"=w4509:dbl, "STATUS"=w4506:string)
                    n2592 = Unbundle(w4527) -> ("CYCLE"=w4515:dbl, "MINS"=w4514:dbl, "STATUS"=w4511:string)
                    n2593 = Unbundle(w4525) -> ("CYCLE"=w4503:dbl, "MINS"=w4502:dbl, "STATUS"=w4501:string)
                    n2594 = Unbundle(w4522) -> ("CYCLE"=w4490:dbl, "MINS"=w4489:dbl, "STATUS"=w4486:string)
                    n2595 = Unbundle(w4523) -> ("CYCLE"=w4495:dbl, "MINS"=w4494:dbl, "STATUS"=w4491:string)
                    n2596 = Unbundle(w4524) -> ("CYCLE"=w4500:dbl, "MINS"=w4499:dbl, "STATUS"=w4496:string)
                    n2597 = Unbundle(w4521) -> ("CYCLE"=w4485:dbl, "MINS"=w4484:dbl, "STATUS"=w4481:string)
                    n2598 = Unbundle(w4520) -> ("CYCLE"=w4480:dbl, "MINS"=w4479:dbl, "STATUS"=w4476:string)
                    n2599 = Unbundle(w4519) -> ("CYCLE"=w4475:dbl, "MINS"=w4474:dbl, "STATUS"=w4471:string)
                    n2600 = Unbundle(w4518) -> ("CYCLE"=w4517:dbl, "MINS"=w4516:dbl, "STATUS"=w4468:string)
                    n2601 = Number To Decimal String(number=w4503) -> (decimal integer string=w4505:string)  [unwired: 1 in]
                    n2602 = Number To Decimal String(number=w4500) -> (decimal integer string=w4498:string)  [unwired: 1 in]
                    n2603 = Number To Decimal String(number=w4495) -> (decimal integer string=w4493:string)  [unwired: 1 in]
                    n2604 = Number To Decimal String(number=w4510) -> (decimal integer string=w4508:string)  [unwired: 1 in]
                    n2605 = Number To Decimal String(number=w4490) -> (decimal integer string=w4488:string)  [unwired: 1 in]
                    n2606 = Number To Decimal String(number=w4515) -> (decimal integer string=w4513:string)  [unwired: 1 in]
                    n2607 = Number To Decimal String(number=w4517) -> (decimal integer string=w4470:string)  [unwired: 1 in]
                    n2608 = Number To Decimal String(number=w4485) -> (decimal integer string=w4483:string)  [unwired: 1 in]
                    n2609 = Number To Decimal String(number=w4480) -> (decimal integer string=w4478:string)  [unwired: 1 in]
                    n2610 = Number To Decimal String(number=w4475) -> (decimal integer string=w4473:string)  [unwired: 1 in]
                    n2611 = Number To Fractional String(number=w4502, precision (6)=w4447) -> (F-format string=w4504:string)  [unwired: 2 in]
                    n2612 = Number To Fractional String(number=w4489, precision (6)=w4447) -> (F-format string=w4487:string)  [unwired: 2 in]
                    n2613 = Number To Fractional String(number=w4499, precision (6)=w4447) -> (F-format string=w4497:string)  [unwired: 2 in]
                    n2614 = Number To Fractional String(number=w4494, precision (6)=w4447) -> (F-format string=w4492:string)  [unwired: 2 in]
                    n2615 = Number To Fractional String(number=w4479, precision (6)=w4447) -> (F-format string=w4477:string)  [unwired: 2 in]
                    n2616 = Number To Fractional String(number=w4484, precision (6)=w4447) -> (F-format string=w4482:string)  [unwired: 2 in]
                    n2617 = Number To Fractional String(number=w4509, precision (6)=w4447) -> (F-format string=w4507:string)  [unwired: 2 in]
                    n2618 = Number To Fractional String(number=w4474, precision (6)=w4447) -> (F-format string=w4472:string)  [unwired: 2 in]
                    n2619 = Number To Fractional String(number=w4514, precision (6)=w4447) -> (F-format string=w4512:string)  [unwired: 2 in]
                    n2620 = Number To Fractional String(number=w4516, precision (6)=w4447) -> (F-format string=w4469:string)  [unwired: 2 in]
                    n2621 = Concatenate Strings(w4446, w4488, w4446, w4487, w4446, w4486) -> (w4462:string)
                    n2622 = Concatenate Strings(w4446, w4483, w4446, w4482, w4446, w4481) -> (w4461:string)
                    n2623 = Concatenate Strings(w4446, w4478, w4446, w4477, w4446, w4476) -> (w4460:string)
                    n2624 = Concatenate Strings(w4446, w4473, w4446, w4472, w4446, w4471) -> (w4459:string)
                    n2625 = Concatenate Strings(w4446, w4470, w4446, w4469, w4446, w4468) -> (w4458:string)
                    n2626 = Concatenate Strings(w4446, w4513, w4446, w4512, w4446, w4511) -> (w4467:string)
                    n2627 = Concatenate Strings(w4446, w4493, w4446, w4492, w4446, w4491) -> (w4463:string)
                    n2628 = Concatenate Strings(w4446, w4508, w4446, w4507, w4446, w4506) -> (w4466:string)
                    n2629 = Concatenate Strings(w4446, w4505, w4446, w4504, w4446, w4501) -> (w4465:string)
                    n2630 = Concatenate Strings(w4446, w4498, w4446, w4497, w4446, w4496) -> (w4464:string)
                    n2631 = Concatenate Strings("]", "\r") -> (w4443:string)
                    n2632 = Concatenate Strings(w4438, w4463, w4443) -> (w4453:string)
                    n2633 = Concatenate Strings(w4440, w4465, w4443) -> (w4455:string)
                    n2634 = Concatenate Strings(w4439, w4464, w4443) -> (w4454:string)
                    n2635 = Concatenate Strings(w4435, w4460, w4443) -> (w4450:string)
                    n2636 = Concatenate Strings(w4436, w4459, w4443) -> (w4451:string)
                    n2637 = Concatenate Strings(w4434, w4461, w4443) -> (w4449:string)
                    n2638 = Concatenate Strings(w4433, w4462, w4443) -> (w4448:string)
                    n2639 = Concatenate Strings(w4437, w4458, w4443) -> (w4452:string)
                    n2640 = Concatenate Strings(w4441, w4466, w4443) -> (w4456:string)
                    n2641 = Concatenate Strings(w4442, w4467, w4443) -> (w4457:string)
                    n2642 = Concatenate Strings(w4457, w4456, w4455, w4454, w4453, w4448, w4449, w4450, w4451, w4452) -> (w4426:string)
                    n2643 = Concatenate Strings("[PANEL/", "DESC/", "CYCLES/", "MINS/", "STATUS]", "\r", w4426) -> (w4425:string)
                    "MAIL REPORT" <- w4425
                    n2644 = global write "Global display 3.vi" "log all"(w4425) -> ()
                  }
                  frame #2 {
                    w4556 = "END"
                    n2645 = local read "mail control"() -> (w4557:string)
                    n2646 = case shown="False" w4552 {
                      tunnel: w4557 -> [w4581 _]
                      tunnel: w4556 -> [w4580 _]
                      tunnel: [w4579 FALSE] -> w4542
                      frame False {
                        n2647 = Equal?(x=w4581, y=w4580) -> (x = y?=w4579:bool)
                      }
                      frame True {
                      }
                    }
                    n2648 = case shown="False" w4558 {
                      tunnel: w4557 -> [w4597 _]
                      tunnel: w4556 -> [w4596 _]
                      tunnel: [w4595 FALSE] -> w4546
                      frame False {
                        n2649 = Equal?(x=w4597, y=w4596) -> (x = y?=w4595:bool)
                      }
                      frame True {
                      }
                    }
                    n2650 = case shown="False" w4555 {
                      tunnel: w4557 -> [w4593 _]
                      tunnel: w4556 -> [w4592 _]
                      tunnel: [w4591 FALSE] -> w4545
                      frame False {
                        n2651 = Equal?(x=w4593, y=w4592) -> (x = y?=w4591:bool)
                      }
                      frame True {
                      }
                    }
                    n2652 = case shown="False" w4553 {
                      tunnel: w4557 -> [w4585 _]
                      tunnel: w4556 -> [w4584 _]
                      tunnel: [w4583 FALSE] -> w4543
                      frame False {
                        n2653 = Equal?(x=w4585, y=w4584) -> (x = y?=w4583:bool)
                      }
                      frame True {
                      }
                    }
                    n2654 = case shown="False" w4554 {
                      tunnel: w4557 -> [w4589 _]
                      tunnel: w4556 -> [w4588 _]
                      tunnel: [w4587 FALSE] -> w4544
                      frame False {
                        n2655 = Equal?(x=w4589, y=w4588) -> (x = y?=w4587:bool)
                      }
                      frame True {
                      }
                    }
                    n2656 = Or(x=w4544, y=w4543) -> (x .or. y?=w4535:bool)
                    n2657 = Or(x=w4546, y=w4545) -> (x .or. y?=w4536:bool)
                    n2658 = Or(x=w4536, y=w4535) -> (x .or. y?=w4531:bool)
                    n2659 = case shown="False" w4548 {
                      tunnel: w4557 -> [w4565 _]
                      tunnel: w4556 -> [w4564 _]
                      tunnel: [w4563 FALSE] -> w4537
                      frame False {
                        n2660 = Equal?(x=w4565, y=w4564) -> (x = y?=w4563:bool)
                      }
                      frame True {
                      }
                    }
                    n2661 = case shown="False" w4547 {
                      tunnel: w4557 -> [w4561 _]
                      tunnel: w4556 -> [w4560 _]
                      tunnel: [w4559 FALSE] -> w4541
                      frame False {
                        n2662 = Equal?(x=w4561, y=w4560) -> (x = y?=w4559:bool)
                      }
                      frame True {
                      }
                    }
                    n2663 = case shown="False" w4549 {
                      tunnel: w4557 -> [w4569 _]
                      tunnel: w4556 -> [w4568 _]
                      tunnel: [w4567 FALSE] -> w4538
                      frame False {
                        n2664 = Equal?(x=w4569, y=w4568) -> (x = y?=w4567:bool)
                      }
                      frame True {
                      }
                    }
                    n2665 = case shown="False" w4551 {
                      tunnel: w4557 -> [w4577 _]
                      tunnel: w4556 -> [w4576 _]
                      tunnel: [w4575 FALSE] -> w4540
                      frame False {
                        n2666 = Equal?(x=w4577, y=w4576) -> (x = y?=w4575:bool)
                      }
                      frame True {
                      }
                    }
                    n2667 = case shown="False" w4550 {
                      tunnel: w4557 -> [w4573 _]
                      tunnel: w4556 -> [w4572 _]
                      tunnel: [w4571 FALSE] -> w4539
                      frame False {
                        n2668 = Equal?(x=w4573, y=w4572) -> (x = y?=w4571:bool)
                      }
                      frame True {
                      }
                    }
                    n2669 = Or(x=w4540, y=w4539) -> (x .or. y?=w4534:bool)
                    n2670 = Or(x=w4538, y=w4537) -> (x .or. y?=w4533:bool)
                    n2671 = Or(x=w4541, y=w4542) -> (x .or. y?=w4529:bool)
                    n2672 = Or(x=w4534, y=w4533) -> (x .or. y?=w4532:bool)
                    n2673 = Or(x=w4531, y=w4532) -> (x .or. y?=w4530:bool)
                    n2674 = Or(x=w4530, y=w4529) -> (x .or. y?=w4528:bool)
                  }
